vi "Spike Detection.vi"(8 "에러 입력(에러 없음)":errorcluster, 9 "Sampling rate":dbl, 10 "Epoch":sgl[][](array[numeric]), 11 "Spike threshold (mV)":dbl) -> (0 "에러 출력":errorcluster, 2 "Number of Spike (1D)":i32[](array[numeric]), 3 "Raster plot":cluster{"location":dbl[], "Sweep":i32[]}[](array[cluster]))   [LabVIEW 2017]
uses:
  <vilib>/addons/Wavelet Analysis/application.llb/WA Multiscale Peak Detection (Array).vi
  <vilib>/addons/_Advanced Signal Processing/NI_AdvSigProcWA.lvlib
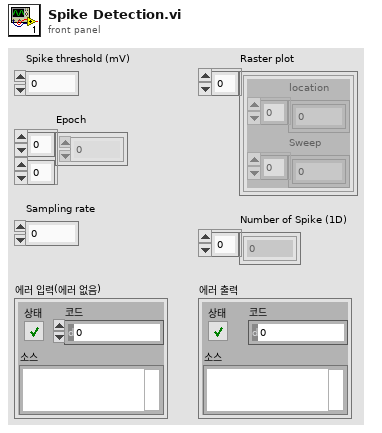
[diagram p1: front panel]
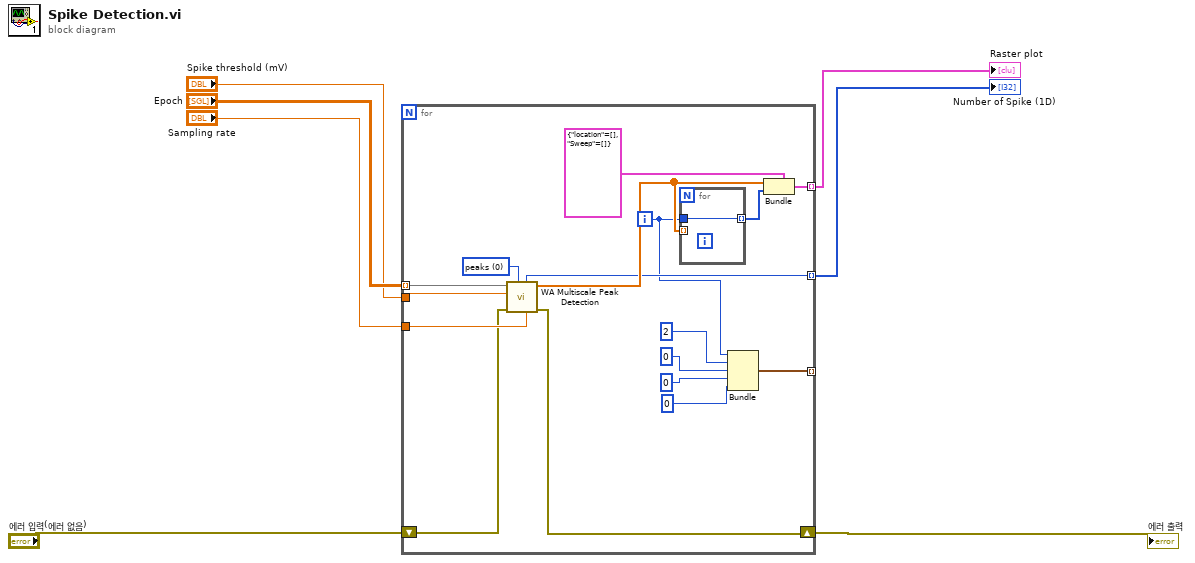
[diagram p0: block diagram]
diagram:
  n1 = for {
    tunnel: "Epoch" -> [w24] mode=indexing
    tunnel: "Spike threshold (mV)" -> [w23]
    tunnel: "Sampling rate" -> [w21]
    tunnel: [w18] -> w6 mode=indexing
    tunnel: [w17] -> w7 mode=indexing
    tunnel: [w10] -> _ mode=indexing
    shift-right: [w8] -> w5
    shift-left: "에러 입력(에러 없음)" -> [w9]
    i -> [w11]
    w22 = u16 0 items=["peaks", "valleys"] ("peaks/valleys")
    n2 = call-poly <vilib>:"WA Multiscale Peak Detection.vi"("sampling rate"=w21, "peaks/valleys"=w22, "error in (no error)"=w9, "threshold"=w23, "signal"=w24) -> ("error out"=w8:errorcluster, "location"=w20:dbl[], "number of peaks"=w17:i32)  [unwired: 2 in, 2 out]
    n3 = for {
      tunnel: w20 -> [_] mode=indexing
      tunnel: w11 -> [w25]
      tunnel: [w25] -> w19 mode=indexing
    }
    n4 = Bundle(w11, u8 2, u8 0, u8 0, u32 0) -> (w10:cluster{i32, u8, u8, u8, u32})  [unwired: 1 in]
    n5 = Bundle(cluster=cluster{"location":dbl[], "Sweep":i32[]} {"location"=[], "Sweep"=[]} ("클러스터"), "location"=w20, "Sweep"=w19) -> (w18:cluster{"location":dbl[], "Sweep":i32[]})
  }
  "Number of Spike (1D)" <- w7
  "Raster plot" <- w6
  "에러 출력" <- w5
